vi "Logitech F310.vi"(6 "error in (no error)":errorcluster, 7 "Deadzone Scale Cluster":cluster{"Scale":dbl, "Deadzone":dbl}, 8 "refnum name":string) -> (0 "Buttons":T2, 1 "D-Pad Buttons":T1, 3 "Right Stick":cluster{"X":dbl, "Y":dbl}, 4 "error out":errorcluster, 5 "Left Stick":cluster{"X":dbl, "Y":dbl})   [LabVIEW 2014]
uses:
  <vilib>/Rock Robotics/WPI/Joystick/WPI_JoystickGetSetRefNum.vi
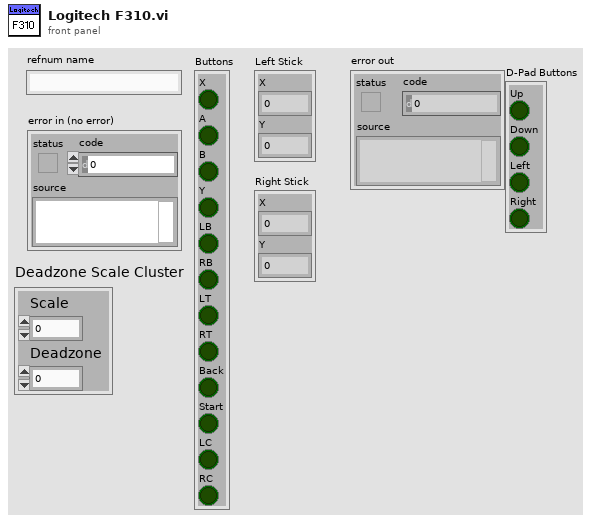
[diagram p1: front panel]
types:
  T1 = cluster{"Up":bool, "Down":bool, "Left":bool, "Right":bool}
  T2 = cluster{"X":bool, "A":bool, "B":bool, "Y":bool, "LB":bool, "RB":bool, "LT":bool, "RT":bool, "Back":bool, "Start":bool, "LC":bool, "RC":bool}
  T3 = typedef "WPI_JoystickDevRef.ctl" = cluster{"Device":T4}
  T4 = typedef "WPI_JoystickDeviceEnum.ctl" = enum16{"USB 0", "USB 1", "USB 2", "USB 3", "USB 4", "USB 5"}
  T5 = cluster{"[0]":dbl, "[1]":dbl, "[2]":dbl, "[3]":dbl}
  T6 = cluster{"Buttons[0]":bool, "Buttons[1]":bool, "Buttons[2]":bool, "Buttons[3]":bool, "Buttons[4]":bool, "Buttons[5]":bool, "Buttons[6]":bool, "Buttons[7]":bool, "Buttons[8]":bool, "Buttons[9]":bool, "Buttons[10]":bool, "Buttons[11]":bool}
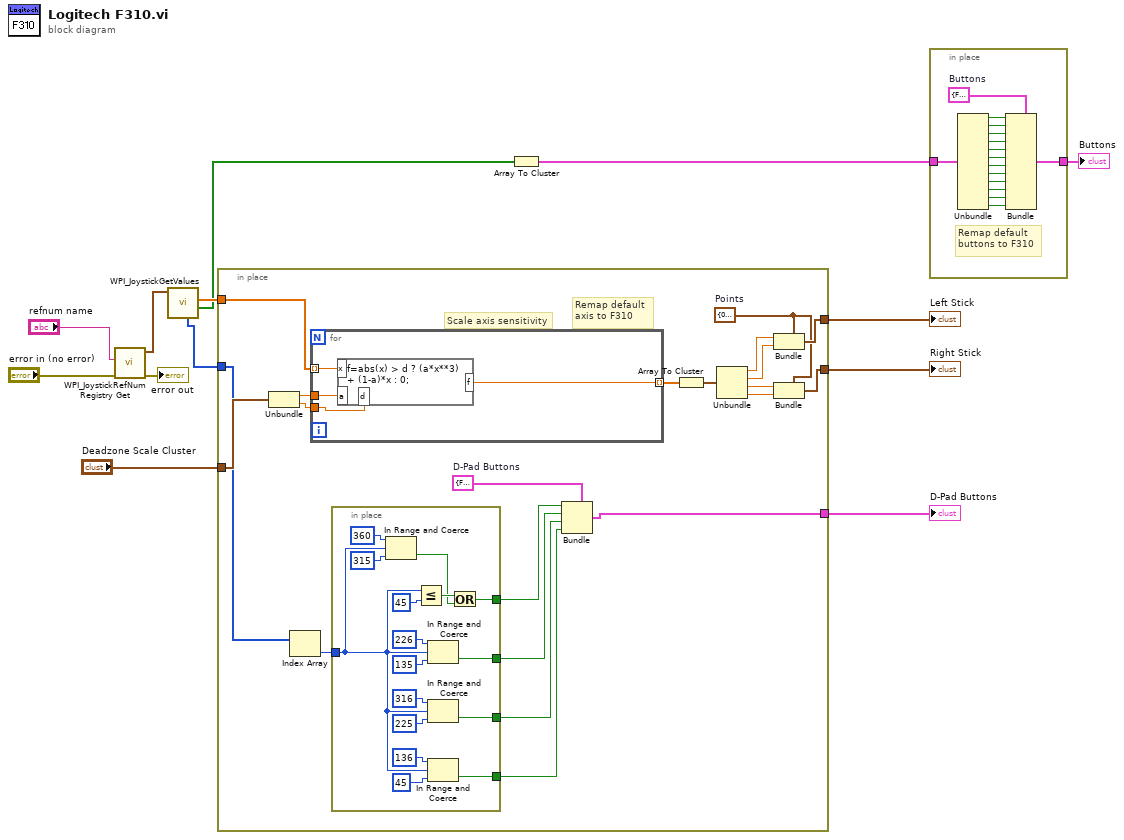
[diagram p0: block diagram]
diagram:
  n1 = call <vilib>:"WPI_JoystickRefNum Registry Get.vi"("error in (no error)"="error in (no error)", "refnum name"="refnum name") -> ("error out"=→"error out":errorcluster, "JoystickDevRef"=w5:T3)  [unwired: 8 in]
  n2 = call <vilib>:"WPI_JoystickGetValues.vi"("JoystickDevRef"=w5) -> ("Buttons"=w2:bool[], "Axes"=w4:dbl[], "POVs"=w1:u16[])  [unwired: 6 in, 2 out]
  n3 = in-place {
    in-place-border: [w34] -> w10
    in-place-border: [w33] -> w9
    in-place-border: [w30] -> w7
    in-place-border: "Deadzone Scale Cluster" -> [w23]
    in-place-border: w4 -> [w20]
    in-place-border: w1 -> [w19]
    w31 = T1 {"Up"=FALSE, "Down"=FALSE, "Left"=FALSE, "Right"=FALSE}  # D-Pad Buttons
    w32 = cluster{"X":dbl, "Y":dbl} {"X"=0.0, "Y"=0.0}  # Points
    # "Remap default\naxis to F310"
    # "Scale axis sensitivity"
    n4 = Unbundle(w23) -> ("Scale"=w22:dbl, "Deadzone"=w21:dbl)
    n5 = Index Array(array=w19) -> (element=w15:u16)  [unwired: 1 in]
    n6 = for {
      tunnel: w20 -> [w54] mode=indexing
      tunnel: [w53] -> w24 mode=indexing
      tunnel: w22 -> [w52]
      tunnel: w21 -> [w51]
      n7 = formula code="f=abs(x) > d ? (a*x**3) + (1-a)*x : 0;"("x"=w54, "a"=w52, "d"=w51) -> ("f"=w53:dbl)
    }
    n8 = in-place {
      in-place-border: [w48] -> w18
      in-place-border: [w45] -> w17
      in-place-border: [w42] -> w16
      in-place-border: w15 -> [w36]
      in-place-border: [w39] -> w14
      n9 = In Range and Coerce(upper limit=u16 360, x=w36, lower limit=u16 315 ("y")) -> (In Range?=w35:bool)  [unwired: 1 out]
      n10 = Less Or Equal?(x=w36, y=u16 45) -> (x <= y?=w49:bool)
      n11 = In Range and Coerce(upper limit=u16 226, x=w36, lower limit=u16 135) -> (In Range?=w42:bool)  [unwired: 1 out]
      n12 = In Range and Coerce(upper limit=u16 316, x=w36, lower limit=u16 225) -> (In Range?=w39:bool)  [unwired: 1 out]
      n13 = In Range and Coerce(upper limit=u16 136, x=w36, lower limit=u16 45) -> (In Range?=w45:bool)  [unwired: 1 out]
      n14 = Or(x=w49, y=w35) -> (x .or. y?=w48:bool)
    }
    n15 = Bundle(cluster=w31, "Up"=w18, "Down"=w16, "Left"=w14, "Right"=w17) -> (w30:T1)
    n16 = Array To Cluster(array=w24) -> (cluster=w25:T5)
    n17 = Unbundle(w25) -> ("[0]"=w29:dbl, "[1]"=w28:dbl, "[2]"=w27:dbl, "[3]"=w26:dbl)
    n18 = Bundle(cluster=w32, "X"=w29, "Y"=w28) -> (w34:cluster{"X":dbl, "Y":dbl})
    n19 = Bundle(cluster=w32, "X"=w27, "Y"=w26) -> (w33:cluster{"X":dbl, "Y":dbl})
  }
  "Left Stick" <- w10
  "Right Stick" <- w9
  "D-Pad Buttons" <- w7
  n20 = Array To Cluster(array=w2) -> (cluster=w3:T6)
  n21 = in-place {
    in-place-border: w3 -> [w69]
    in-place-border: [w55] -> w8
    w68 = T2 {"X"=FALSE, "A"=FALSE, "B"=FALSE, "Y"=FALSE, "LB"=FALSE, "RB"=FALSE, "LT"=FALSE, "RT"=FALSE, "Back"=FALSE, "Start"=FALSE, "LC"=FALSE, "RC"=FALSE}  # Buttons
    # "Remap default\nbuttons to F310"
    n22 = Unbundle(w69) -> ("Buttons[0]"=w67:bool, "Buttons[1]"=w66:bool, "Buttons[2]"=w65:bool, "Buttons[3]"=w64:bool, "Buttons[4]"=w63:bool, "Buttons[5]"=w62:bool, "Buttons[6]"=w61:bool, "Buttons[7]"=w60:bool, "Buttons[8]"=w59:bool, "Buttons[9]"=w58:bool, "Buttons[10]"=w57:bool, "Buttons[11]"=w56:bool)
    n23 = Bundle(cluster=w68, "X"=w67, "A"=w66, "B"=w65, "Y"=w64, "LB"=w63, "RB"=w62, "LT"=w61, "RT"=w60, "Back"=w59, "Start"=w58, "LC"=w57, "RC"=w56) -> (w55:T2)
  }
  "Buttons" <- w8
